vi "TestExec.Setup Test Exec Config.vi"(8 "error in (no error)":errorcluster, 9 "Over Write":bool, 10 "Station App Exe Path":path, 11 "Application Name":string) -> (0 "error out":errorcluster, 2 "Modified":bool)   [LabVIEW 2019]
uses:
  <vilib>/Utility/config.llb/Write Key (String).vi
  <vilib>/KATE/Files/File Utils.lvlib
  <vilib>/Utility/config.llb/NI_LVConfig.lvlib
panel:
  # "This VI copies a file or folder from one location to another on the PC.\nFiles/Folders will only be copied of they do not exist."
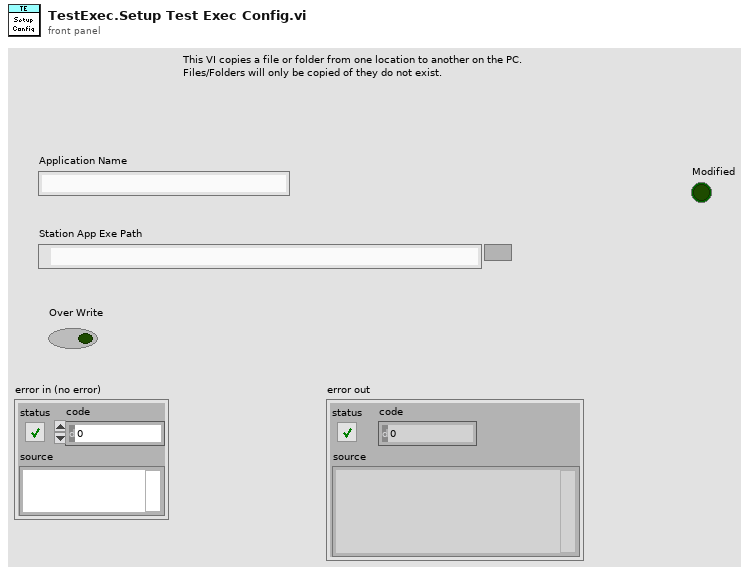
[diagram p1: front panel]
types:
  T1 = typedef "NI_LVConfig.lvlib/Config Data RefNum.ctl" = refnum<k1>
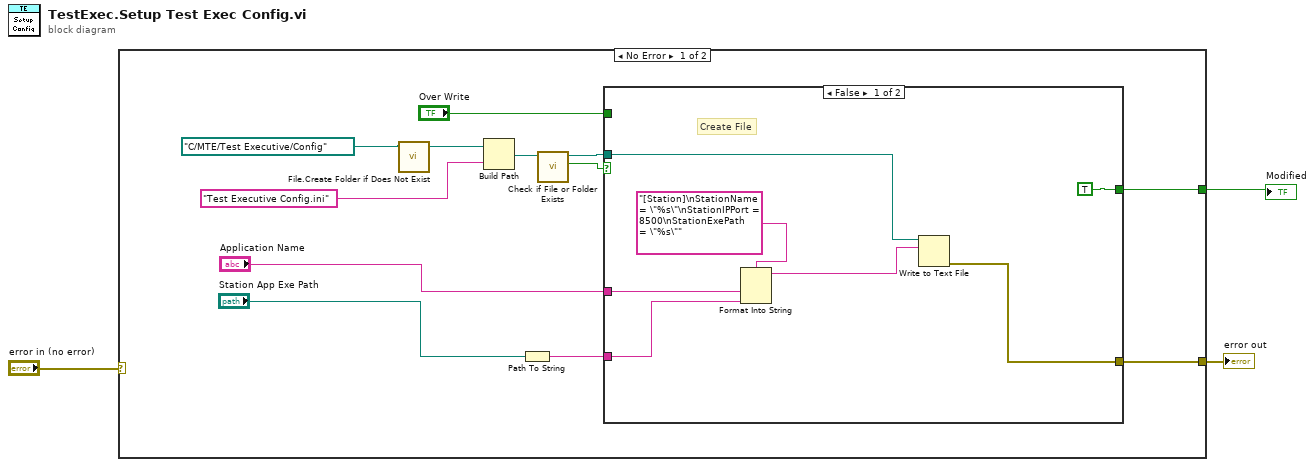
[diagram p0: block diagram]
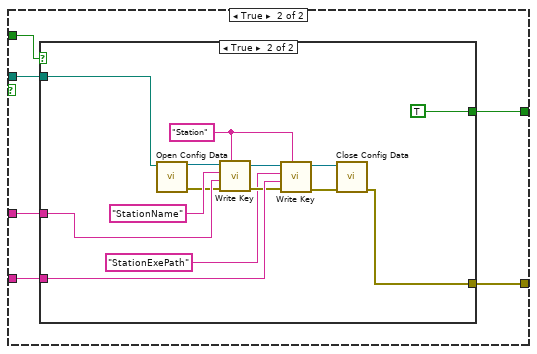
[diagram p2: hidden frame]
diagram:
  n1 = case shown="No Error" "error in (no error)" {
    selector: "error in (no error)" -> [_ w43]
    tunnel: [w8 w43] -> w2
    tunnel: [w4 _] -> w1
    frame No Error {
      n2 = call <vilib>:"File.Create Folder if Does Not Exist.vi"("Path"=path "C:/MTE/Test Executive/Config") -> ("Dup Path"=w14:path)  [unwired: 8 in, 2 out]
      n3 = Build Path(base path=w14, name or relative path="Test Executive Config.ini") -> (appended path=w12:path)
      n4 = Path To String(path="Station App Exe Path") -> (string=w6:string)
      n5 = call <vilib>:"Check if File or Folder Exists.vi"("path"=w12) -> ("file or folder exists?"=w11:bool, "dup path"=w10:path)  [unwired: 8 in, 1 out]
      n6 = case shown="False" w11 {
        tunnel: w10 -> [w20 w28]
        tunnel: w6 -> [w17 w26]
        tunnel: "Application Name" -> [w21 w27]
        tunnel: [w18 w25] -> w8
        tunnel: "Over Write" -> [_ w24]
        tunnel: [TRUE w23] -> w4
        frame False {
          # "Create File"
          n7 = Format Into String(format string="[Station]\nStationName = \"%s\"\nStationIPPort = 8500\nStationExePath = \"%s\"", w21, w17) -> (resulting string=w19:string)  [unwired: 2 in, 1 out]
          n8 = Write to Text File(file (use dialog)=w20, text=w19) -> (error out=w18:errorcluster)  [unwired: 2 in, 2 out]
        }
        frame True {
          n9 = case shown="True" w24 {
            tunnel: w28 -> [_ w42]
            tunnel: w27 -> [_ w39]
            tunnel: w26 -> [_ w38]
            tunnel: [_ w30] -> w25
            tunnel: [_ TRUE] -> w23
            frame False {
            }
            frame True {
              w34 = "Station"
              n10 = call <vilib>:"Open Config Data.vi"("configuration file path"=w42) -> ("error out"=w35:errorcluster, "refnum"=w41:T1)  [unwired: 8 in, 1 out]
              n11 = call-poly <vilib>:"Write Key.vi"("section"=w34, "error in (no error)"=w35, "value"=w39, "key"="StationName", "refnum"=w41) -> ("error out"=w36:errorcluster, "refnum out"=w37:T1)  [unwired: 4 in, 1 out]
              n12 = call-poly <vilib>:"Write Key.vi"("section"=w34, "error in (no error)"=w36, "value"=w38, "key"="StationExePath", "refnum"=w37) -> ("error out"=w32:errorcluster, "refnum out"=w31:T1)  [unwired: 4 in, 1 out]
              n13 = call <vilib>:"Close Config Data.vi"("error in (no error)"=w32, "refnum"=w31) -> ("error out"=w30:errorcluster)  [unwired: 8 in, 1 out]
            }
          }
        }
      }
    }
    frame Error {
    }
  }
  "error out" <- w2
  "Modified" <- w1
